vi "Init.vi"(8 "error in (no error)":errorcluster, 10 "Configuration":T1={"Cycle Period"=0.0, "Ismatech"={"VISA resource name"="", "Simulated?"=FALSE, "Pump Number"=1.0, "Reverse?"=FALSE}, "Masterflex"={"VISA resource name"="", "Simulated?"=FALSE, "Pump Number"=1.0, "Reverse?"=FALSE}, "Mettler"={"VISA resource name"="", "Simulated?"=FALSE}, "Bronkhorst M13 Flow Meter"={"VISA resource name"="", "Simulated?"=FALSE}, "PID 2 Parameters"={"Input Device"=enum."Flowmeter", "Output Device"=enum."Ismatec ISM 831C", "Setpoint"=0.0, "PID gains"={"proportional gain (Kc)"=1.0, "integral time (Ti, min)"=0.01, "derivative time (Td, min)"=0.0}}, "Manual Entry"=0.0, "Auto?"=TRUE, "VICI Settings"={"VISA resource name"="", "Simulated?"=FALSE, "Pump Number"=0.0, "Reverse?"=FALSE}, "output range"={"output high"=100.0, "output low"=0.0}} {"output range"."output low" min=0.0 max=100.0 format="%.2f"; "output range"."output high" format="%.2f"; "VICI Settings"."Pump Number" min=1.0 max=20.0 step=1.0; "PID 2 Parameters"."PID gains"."derivative time (Td, min)" format="%.3f"; "PID 2 Parameters"."PID gains"."integral time (Ti, min)" format="%.3f"; "PID 2 Parameters"."PID gains"."proportional gain (Kc)" format="%.3f"; "Masterflex"."Pump Number" min=1.0 max=20.0 step=1.0; "Ismatech"."Pump Number" min=1.0 max=20.0 step=1.0}, 11 "Hardware in":refnum<class "Hardware.lvclass">) -> (0 "error out":errorcluster, 3 "Hardware out":refnum<class "Hardware.lvclass">)   [LabVIEW 2018, in "Hardware.lvclass"]
uses:
  Hardware.lvclass
  Feed Module/Controls/Feed Module Settings Cluster.ctl
  Ismatec ISM 831C/Controls/Ismatech Settings Cluster.ctl
  Masterflex 7550-30/Controls/Settings Cluster.ctl
  Mettler Toledo/Controls/Settings Cluster.ctl
  Bronkhorst M13 Flow Meter/Settings Cluster.ctl
  Measure Instrument/PID 2 Parameters Cluster.ctl
  Measure Instrument/PID Input Enum.ctl
  Measure Instrument/PID 2 Output Enum.ctl
  VICI M50/VICI Settings.ctl
  Feed Module/Feed Module.lvlib
  Ismatec ISM 831C/Ismatec ISM 831C.lvlib
  Masterflex 7550-30/Masterflex 7550-30.lvlib
  Mettler Toledo/Mettler Toledo.lvlib
  Bronkhorst M13 Flow Meter/Bronkhorst M13 Flow Meter.lvlib
panel:
  # "Output Instruments"
  # "Input Instruments"
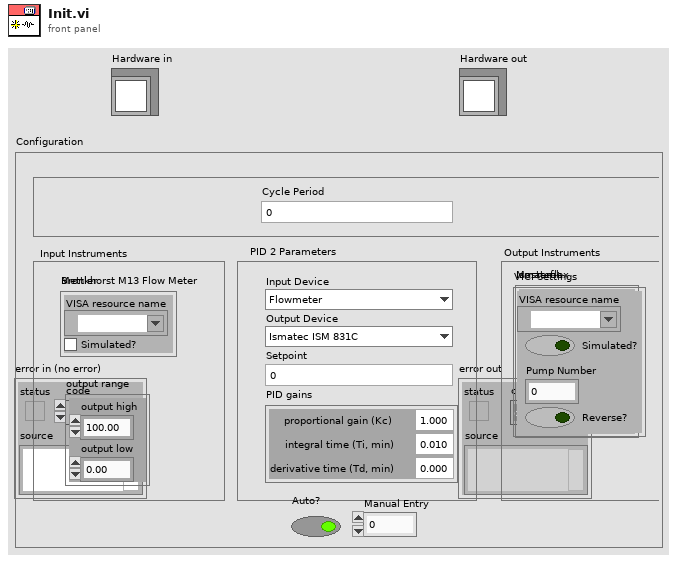
[diagram p1: front panel]
types:
  T1 = typedef "Feed Module.lvlib/Feed Module Settings Cluster.ctl" = cluster{"Cycle Period":dbl, "Ismatech":T2, "Masterflex":T3, "Mettler":T4, "Bronkhorst M13 Flow Meter":T5, "PID 2 Parameters":T6, "Manual Entry":dbl, "Auto?":bool, "VICI Settings":T9, "output range":cluster{"output high":dbl, "output low":dbl}}
  T2 = typedef "Ismatec ISM 831C.lvlib/Ismatech Settings Cluster.ctl" = cluster{"VISA resource name":refnum<visa-resource-name>, "Simulated?":bool, "Pump Number":dbl, "Reverse?":bool}
  T3 = typedef "Masterflex 7550-30.lvlib/Settings Cluster.ctl" = cluster{"VISA resource name":refnum<visa-resource-name>, "Simulated?":bool, "Pump Number":dbl, "Reverse?":bool}
  T4 = typedef "Mettler Toledo.lvlib/Settings Cluster.ctl" = cluster{"VISA resource name":refnum<visa-resource-name>, "Simulated?":bool}
  T5 = typedef "Bronkhorst M13 Flow Meter.lvlib/Settings Cluster.ctl" = cluster{"VISA resource name":refnum<visa-resource-name>, "Simulated?":bool}
  T6 = typedef "PID 2 Parameters Cluster.ctl" = cluster{"Input Device":T7, "Output Device":T8, "Setpoint":dbl, "PID gains":cluster{"proportional gain (Kc)":dbl, "integral time (Ti, min)":dbl, "derivative time (Td, min)":dbl}}
  T7 = typedef "PID Input Enum.ctl" = enum16{"Default", "Flowmeter", "Scale Rate of Change"}
  T8 = typedef "PID 2 Output Enum.ctl" = enum16{"Default", "Ismatec ISM 831C", "Masterflex 7550-30", "VICI M50"}
  T9 = typedef "VICI Settings.ctl" = cluster{"VISA resource name":refnum<visa-resource-name>, "Simulated?":bool, "Pump Number":dbl, "Reverse?":bool}
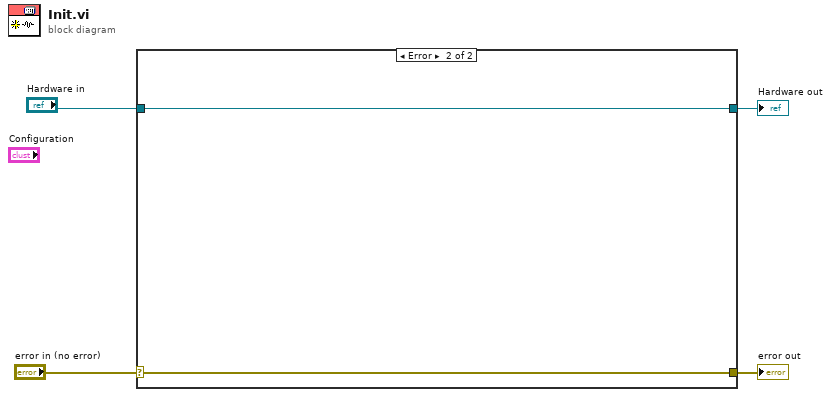
[diagram p0: block diagram]
diagram:
  n1 = case shown="Error" "error in (no error)" {
    selector: "error in (no error)" -> [w6 w8]
    tunnel: [w6 w8] -> w3
    tunnel: [w5 w7] -> w2
    tunnel: "Hardware in" -> [w5 w7]
    frame No Error {
      # "Wire the error cluster across even in the \"No Error\"\ncase so that warnings get propagated."
    }
    frame Error {
    }
  }
  "error out" <- w3
  "Hardware out" <- w2
